vi "Drive Away from Obstacle of Tank1Attck.vi"(4 "angle":dbl, 5 "max reverse velocity (m/s)":dbl, 6 "Find":bool, 7 "max angular velocity (rad/s)":dbl=1.0, 8 "error in (no error)":errorcluster, 9 "Tank1":dbl[](array[numeric]), 10 "Tank2":dbl[](array[numeric]), 11 "gap":T1) -> (0 "error out":errorcluster, 2 "steering frame velocity":dbl[](array[numeric]))   [LabVIEW 2012]
doc: "Sets the steering frame velocity so that the robot moves in reverse and rotates towards the gap."
uses:
  <vilib>/robotics/Obstacle Avoidance/Simple Vector Field Histogram/Gap Description.ctl
  <vilib>/imath/engines/lvmath2/RunTimeEngine/ErrorHandling/NIMS_Finalize Error.vi
  <vilib>/robotics/Obstacle Avoidance/Simple Vector Field Histogram/NI_Robotics_Simple Vector Field Histogram.lvlib
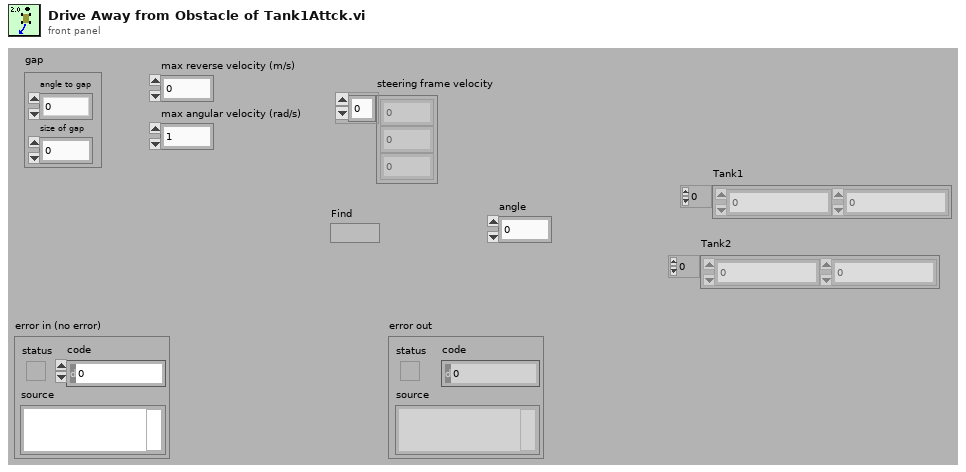
[diagram p1: front panel]
types:
  T1 = typedef "NI_Robotics_Simple Vector Field Histogram.lvlib/Gap Description.ctl" = cluster{"angle to gap":dbl, "size of gap":dbl}
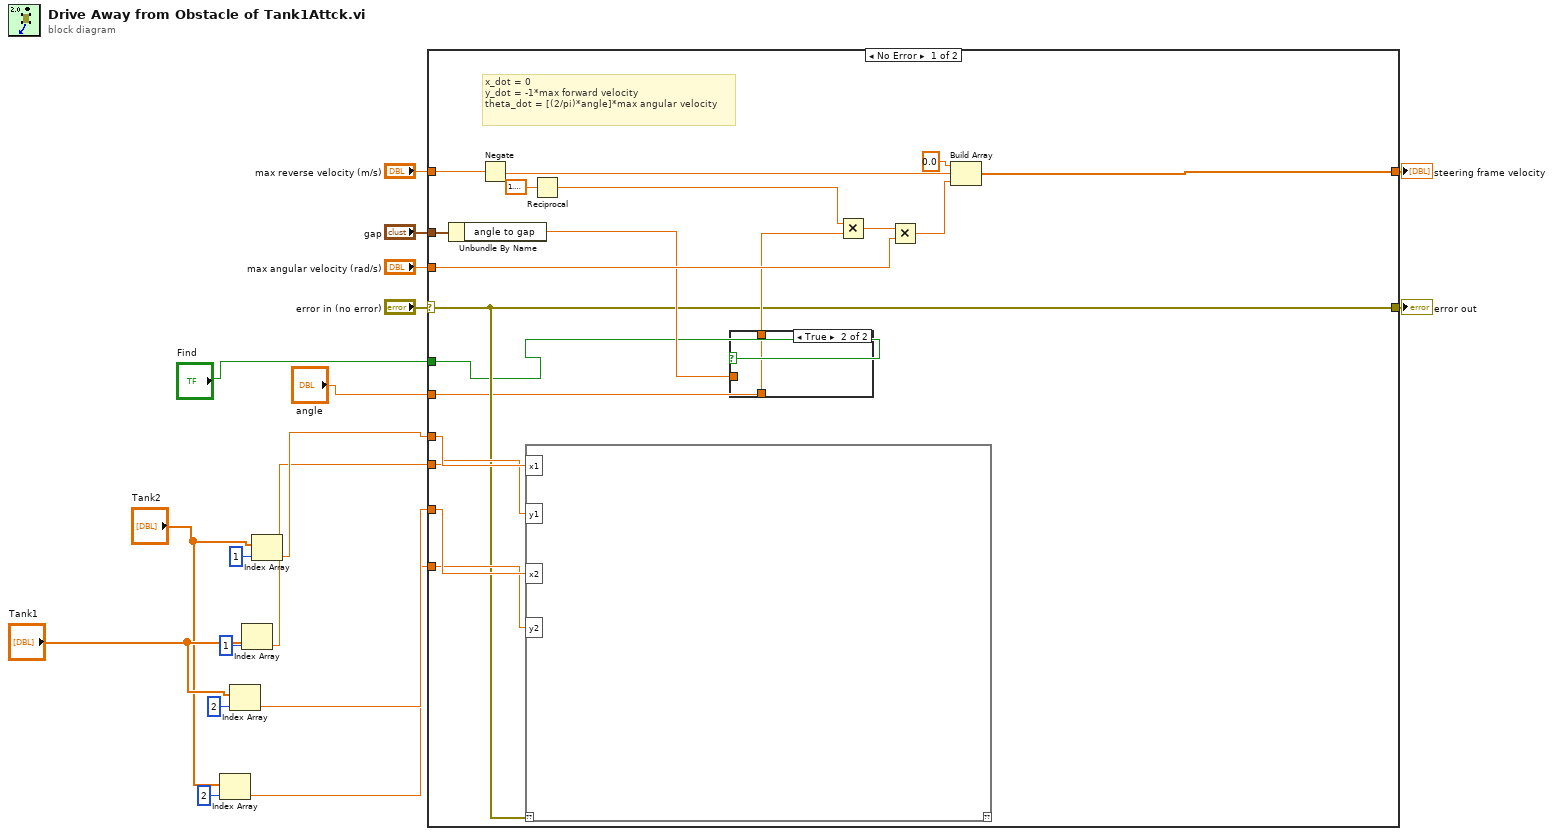
[diagram p0: block diagram]
diagram:
  n1 = Index Array(array="Tank2", index=2) -> (element=w5:dbl)
  n2 = Index Array(array="Tank1", index=2) -> (element=w6:dbl)
  n3 = Index Array(array="Tank1", index=1) -> (element=w7:dbl)
  n4 = Index Array(array="Tank2", index=1) -> (element=w8:dbl)
  n5 = case shown="No Error" "error in (no error)" {
    selector: "error in (no error)" -> [w21 w50]
    tunnel: "gap" -> [w37 _]
    tunnel: [w21 w50] -> w16
    tunnel: "max reverse velocity (m/s)" -> [w34 _]
    tunnel: "max angular velocity (rad/s)" -> [w29 _]
    tunnel: [w35 _] -> w13
    tunnel: w8 -> [w25 _]
    tunnel: w7 -> [w24 _]
    tunnel: w6 -> [w23 _]
    tunnel: w5 -> [w22 _]
    tunnel: "Find" -> [w20 _]
    tunnel: "angle" -> [w19 _]
    frame No Error {
      # "x_dot = 0\ny_dot = -1*max forward velocity\ntheta_dot = [(2/pi)*angle]*max angular velocity"
      n6 = Unbundle By Name(w37) -> ("angle to gap"=w27:dbl)
      n7 = Negate(x=w34) -> (-x=w33:dbl)
      n8 = mathscript code="1"("??"=w21, "x1"=w25, "y1"=w24, "x2"=w23, "y2"=w22) -> ()  [unwired: 1 out]
      n9 = Reciprocal(x=1.5707963267948966) -> (1/x=w31:dbl)
      n10 = case shown="True" w20 {
        tunnel: w27 -> [w48 _]
        tunnel: w19 -> [_ w49]
        tunnel: [w48 w49] -> w26
        frame False {
        }
        frame True {
        }
      }
      n11 = Multiply(x=w31, y=w26) -> (x*y=w30:dbl)
      n12 = Multiply(x=w30, y=w29) -> (x*y=w28:dbl)
      n13 = Build Array(0.0 ("element"), w33, w28) -> (w35:dbl[])
    }
    frame Error {
    }
  }
  "error out" <- w16
  "steering frame velocity" <- w13
